vi "Get Class.vi"() -> ()   [LabVIEW 2015]
doc: "<b> </b> <b> </b>\n©2016 Q Software Innovations, LLC (QSI)\nwritten by Quentin Alldredge\nproduced in LabVIEW 2015"
panel:
  out "Class Name":string
  in  "Numeric":i32
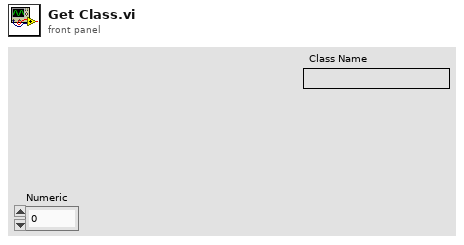
[diagram p1: front panel]
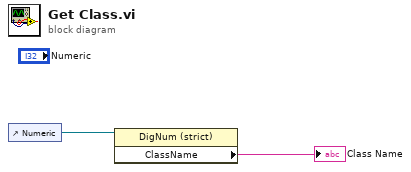
[diagram p0: block diagram]
diagram:
  n1 = control-ref of="Numeric"() -> (w1:refnum<vi>)
  n2 = property class="DigNum (strict)"(reference=w1) -> ("ClassName"=→"Class Name":string)  [unwired: 1 in, 2 out]
